vi "PH_Stepmotor_BaseClass.Axis DIM update Settings Service.vi"(3 "error in (no error)":errorcluster, 4 "Axis Settings":T2={"Sign change"=FALSE, "Width"=0.0, "Calibration"=0.0, "Unit"="Steps", "Motor Type"=enum."Unspecific", "Unit Width"="", "Unit CF"=""}, 5 "Axis DIM IDs":T1) -> (0 "error out":errorcluster)   [LabVIEW 2014, in "PH_Stepmotor_BaseClass.lvlib"]
uses:
  PH_Stepmotor_BaseClass.lvlib
  PH_Stepmotor_BaseClass.Axis Settings.ctl
  PH_Stepmotor_BaseClass.Motor Type.ctl
  PH_Stepmotor_BaseClass.Axis DIM Service IDs.ctl
  lib.lib/DimLVEvent/LVDimInterface/LVDimInterface.lvlib
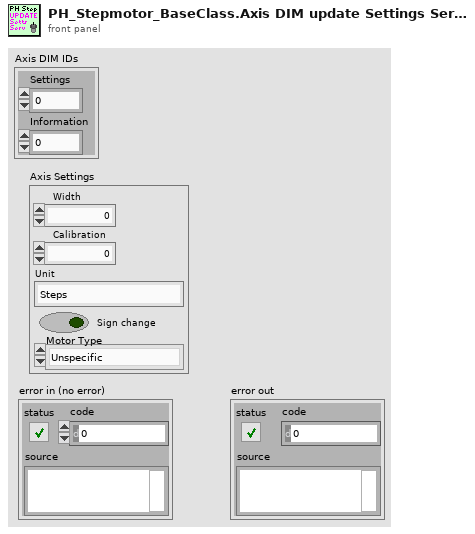
[diagram p1: front panel]
types:
  T1 = typedef "PH_Stepmotor_BaseClass.lvlib/PH_Stepmotor_BaseClass.Axis DIM Service IDs.ctl" = cluster{"Settings":i32, "Information":i32}
  T2 = typedef "PH_Stepmotor_BaseClass.lvlib/PH_Stepmotor_BaseClass.Axis Settings.ctl" = cluster{"Sign change":bool, "Width":dbl, "Calibration":dbl, "Unit":string, "Motor Type":T3, "Unit Width":string, "Unit CF":string}
  T3 = typedef "PH_Stepmotor_BaseClass.lvlib/PH_Stepmotor_BaseClass.Motor Type.ctl" = enum16{"Unspecific", "OWIS 49.120.2633", "OWIS 49.060.1033", "OWIS 43.040.2558", "Diamond Motion 2200 series", "OWIS 49.120.266B.MV6", "Calorimeter", "Linear Stage 1", "MICOS VT-80", "MICOS VT-80 S", "Standa Rotstage nt0.95A", "PUF RA 320.200", "PUF RA 800.200", "PUF RA 800.400", "PUF RA 400.50", "1324.nn.800.50", "1324.n9c.800.50", "1324.nn.320.200", "1324.nn.400.200", "1324.nn.800.200", "1324.nn.400.50", "1324.8c9c.800.50", "1324.8c9c.400.200"}
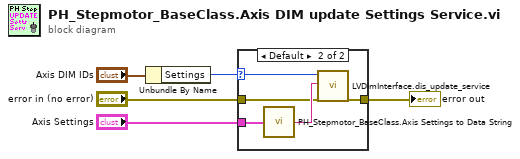
[diagram p0: block diagram]
diagram:
  n1 = Unbundle By Name("Axis DIM IDs") -> ("Settings"=w1:i32)
  n2 = case shown="Default" w1 {
    selector: w1 -> [_ w8]
    tunnel: [w6 w11] -> w2
    tunnel: "Axis Settings" -> [_ w10]
    tunnel: "error in (no error)" -> [w6 w7]
    frame -1 {
    }
    frame Default {
      n3 = call "PH_Stepmotor_BaseClass.Axis Settings to Data String.vi"("Axis Settings"=w10) -> ("Data String"=w9:string)
      n4 = call "LVDimInterface.dis_update_service.vi"("my_serviceID"=w8, "data"=w9, "error in (no error)"=w7) -> ("error out"=w11:errorcluster)  [unwired: 14 in, 2 out]
    }
  }
  "error out" <- w2
